vi "Sub Initialize.vi"(8 "error in (no error)":errorcluster, 11 "Format Resonances in":refnum<class "Format Resonances.lvclass">) -> (0 "error out":errorcluster, 2 "Initialize Result":refnum<class "Acquired Result.lvclass">, 3 "Format Resonances out":refnum<class "Format Resonances.lvclass">)   [LabVIEW 2016, in "Format Resonances.lvclass"]
uses:
  Format Resonances.lvclass
  C:/github/LabActor/Process Object/Process Object.lvclass
  NHMFL_Core/Libraries/Instruments/Results/Acquired Result/Acquired Result.lvclass
  Process Object/Process Object.lvclass/Process Object.ctl
  Process Object/Write Broadcaster name.vi
  Read Elastic Moduli Configuration.vi
  Process Object/Process Object.lvclass
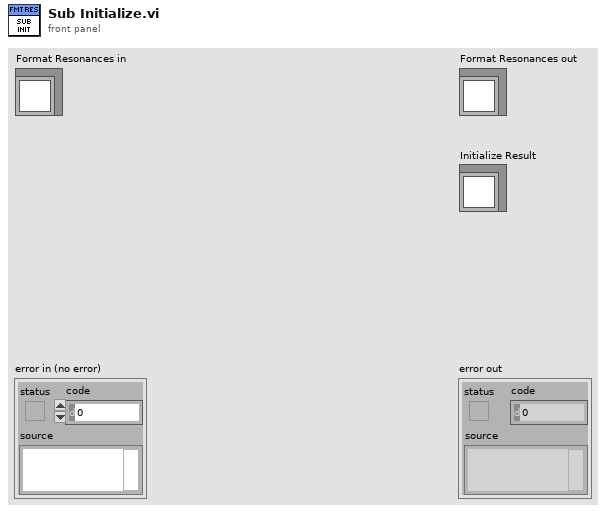
[diagram p1: front panel]
types:
  T1 = typedef "Format Resonances Configuration.ctl" = cluster{"Output header ":string, "rusin\n.dat":enum16{"NONE", "With header", "Without header"}, "Resonance detector module name":string, "Save sp*.dat":bool}
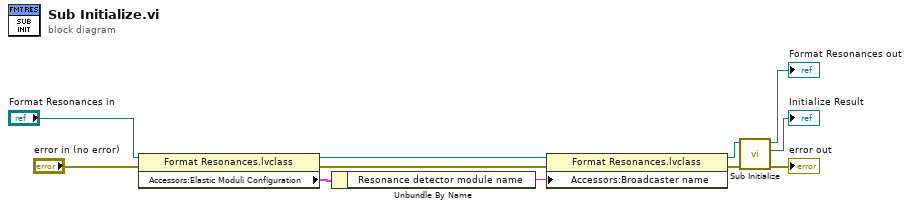
[diagram p0: block diagram]
diagram:
  n1 = property class="Format Resonances.lvclass"(reference="Format Resonances in", error in="error in (no error)") -> (reference out=w8:refnum<class "Format Resonances.lvclass">, error out=w6:errorcluster, "Accessors:Elastic Moduli Configuration"=w10:T1)
  n2 = Unbundle By Name(w10) -> ("Resonance detector module name"=w7:string)
  n3 = property class="Format Resonances.lvclass"(reference=w8, error in=w6, "Accessors:Broadcaster name"=w7) -> (reference out=w5:refnum<class "Format Resonances.lvclass">, error out=w3:errorcluster)
  n4 = call-parent "Sub Initialize.vi"("error in (no error)"=w3, "Measure Object in"=w5) -> ("error out"=→"error out":errorcluster, "Initialize Result"=→"Initialize Result":refnum<class "Acquired Result.lvclass">, "Measure Object out"=→"Format Resonances out":refnum<class "Format Resonances.lvclass">)  [unwired: 7 in]
